vi "led3.vi"() -> ()   [LabVIEW 2014]
panel:
  out "led3":bool
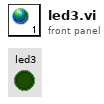
[diagram p1: front panel]
diagram:
